vi "IP_GetList.vi"(8 "Error In":errorcluster caption="Entrée d'erreur", 11 "MustContain":string) -> (0 "Error Out":errorcluster caption="Sortie d'erreur", 3 "IP_List":string[](array[string]))   [LabVIEW 2013]
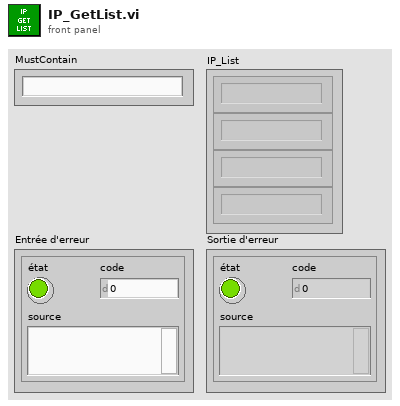
[diagram p1: front panel]
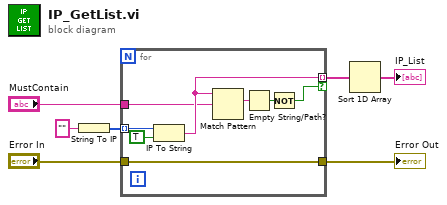
[diagram p0: block diagram]
diagram:
  n1 = String To IP(1:"" ("nom")) -> (0:w7:u32[])
  n2 = for {
    tunnel: w7 -> [w15] mode=indexing
    tunnel: [w13] -> w2 mode=indexing if=w9
    tunnel: "MustContain" -> [w8]
    tunnel: [w12] -> w4
    tunnel: "Error In" -> [w12]
    n3 = IP To String(1:TRUE ("notation à points ? (F)"), 2:w15) -> (0:w13:string)
    n4 = Match Pattern(string=w13, regular expression=w8) -> (match substring=w11:string)  [unwired: 1 in, 3 out]
    n5 = Empty String/Path?(string/path=w11) -> (empty?=w10:bool)
    n6 = Not(x=w10) -> (.not. x?=w9:bool)
  }
  "Error Out" <- w4
  n7 = Sort 1D Array(array=w2) -> (sorted array=→"IP_List":string[])
